vi "WASD Keyboard Drive.vi"() -> (0 "Y-Axis":dbl, 1 "X-Axis":dbl, 2 "key":T1(ring))   [LabVIEW 2012]
uses:
  <vilib>/Utility/inputDevices.llb/keyboardAcquire.vi
  <vilib>/Utility/inputDevices.llb/mouseAcquire.vi
panel:
  in  "Scrolling Down Constant":dbl
  out "Scrolling Down":dbl
  out "button 4":bool
  out "button 3":bool
  out "button 2":bool
  out "button 1":bool
  out "Horizontal Max":dbl
  in  "Scrolling Up Constant":dbl
  out "Vertical":dbl
  out "Horizontal":dbl
  out "Scrolling Up":dbl
  in  "mouse":bool
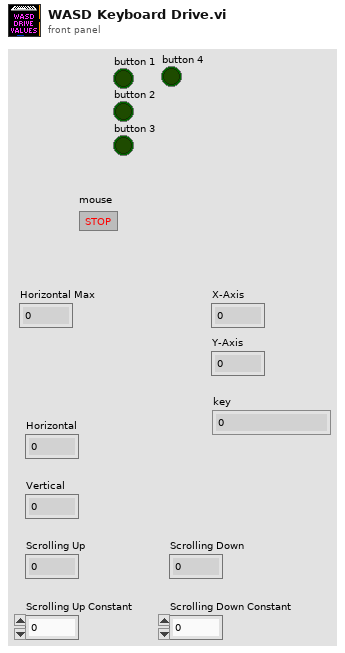
[diagram p1: front panel]
types:
  T1 = enum16{"0", "1", "2", "3", "4", "5", "6", "7", "8", "9", "A", "B", "C", "D", "E", "F", "G", "H", "I", "J", "K", "L", "M", "N", "O", "P", "Q", "R", "S", "T", "U", "V", "W", "X", "Y", "Z", "F1", "F2", "F3", "F4", "F5", "F6", "F7", "F8", "F9", "F10", "F11", "F12", "F13", "F14", "F15", "ADD", "BACK", "BACKSLASH", "CAPITAL", "COMMA", "DECIMAL", "DELETE", "DIVIDE", "DOWN", "END", "EQUALS", "ESCAPE", "GRAVE (`)", "HOME", "INSERT", "LBRACKET", "LCONTROL", "LEFT", "L ALT", "LSHIFT", "LWIN", "MINUS", "MULTIPLY", "NEXT", "NUMLOCK", "NUMPAD_0", "NUMPAD_1", "NUMPAD_2", "NUMPAD_3", "NUMPAD_4", "NUMPAD_5", "NUMPAD_6", "NUMPAD_7", "NUMPAD_8", "NUMPAD_9", "PAUSE", "PERIOD", "PRIOR (PG UP)", "RBRACKET", "RCONTROL", "RETURN", "RIGHT", "R ALT", "RSHIFT", "RWIN", "SCROLL", "SEMICOLON", "SLASH", "SPACE", "SUBTRACT", "TAB", "UP", "ENTER (num pad)", "' (quote)"}
  T2 = cluster{"Horizontal":i32, "Vertical":i32, "Scrolling":i32}
  T3 = cluster{"button 1":bool, "button 2":bool, "button 3":bool, "button 4":bool}
  T4 = enum16{"0", "1", "2", "3", "4", "5", "6", "7", "8", "9", "A", "B", "C", "D", "E", "F", "G", "H", "I", "J", "K", "L", "M", "N", "O", "P", "Q", "R", "S", "T", "U", "V", "W", "X", "Y", "Z", "F1", "F2", "F3", "F4", "F5", "F6", "F7", "F8", "F9", "F10", "F11", "F12", "F13", "F14", "F15", "ADD", "BACK", "BACKSLASH", "CAPITAL", "COMMA", "DECIMAL", "DELETE", "DIVIDE", "DOWN", "END", "EQUALS", "ESCAPE", "GRAVE (`)", "HOME", "INSERT", "LBRACKET", "LCONTROL", "LEFT", "L ALT", "LSHIFT", "LWIN", "MINUS", "MULTIPLY", "NEXT", "NUMLOCK", "NUMPAD_0", "NUMPAD_1", "NUMPAD_2", "NUMPAD_3", "NUMPAD_4", "NUMPAD_5", "NUMPAD_6", "NUMPAD_7", "NUMPAD_8", "NUMPAD_9", "PAUSE", "PERIOD", "PRIOR (PG UP)", "RBRACKET", "RCONTROL", "RETURN", "RIGHT", "R ALT", "RSHIFT", "RWIN", "SCROLL", "SEMICOLON", "SLASH", "SPACE", "SUBTRACT", "TAB", "UP", "ENTER (num pad)", "' (quote)"}[]
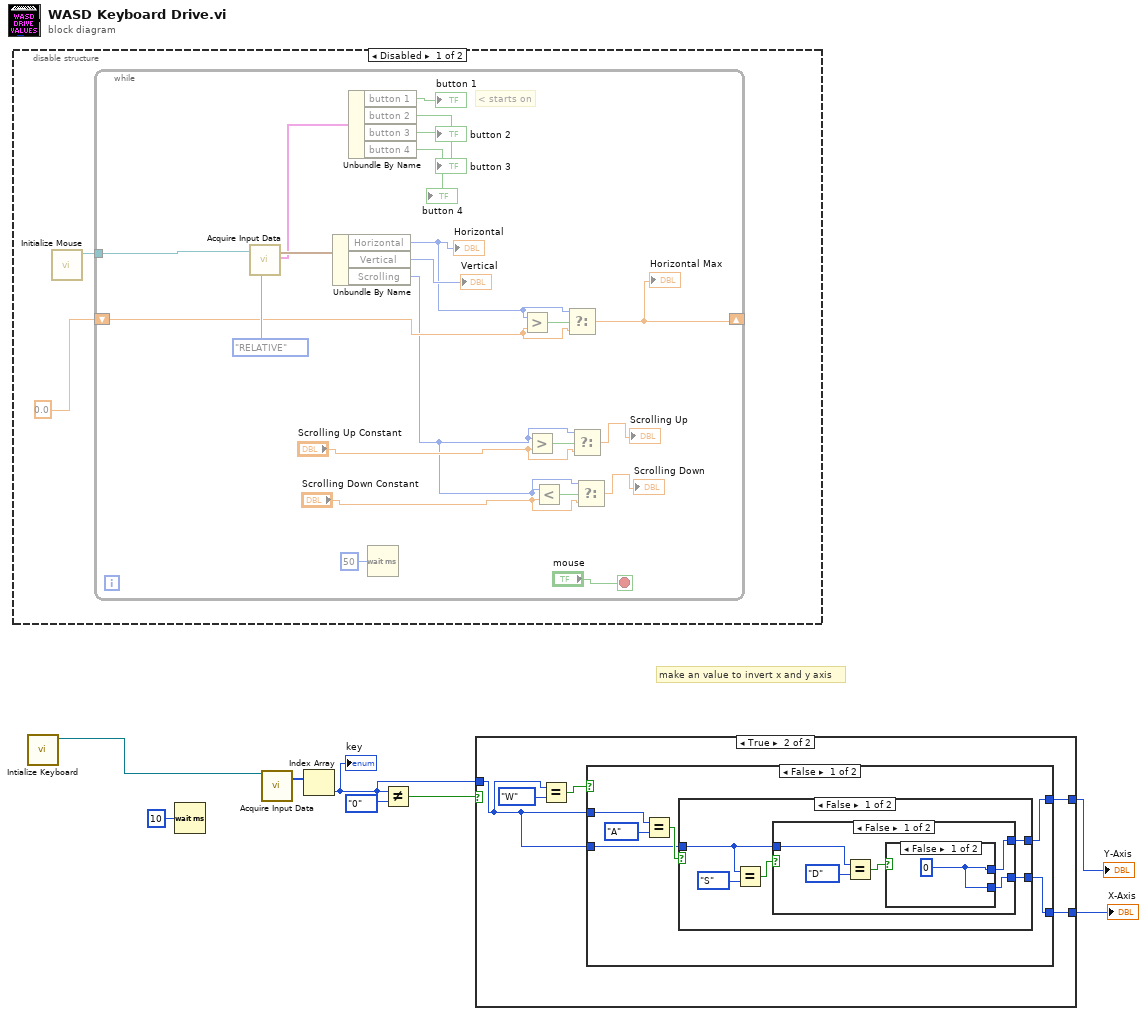
[diagram p0: block diagram]
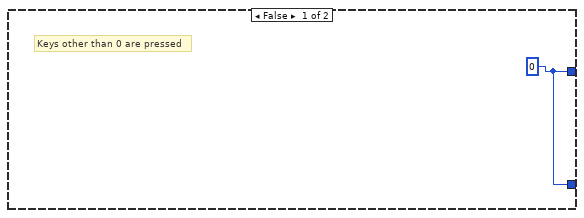
[diagram p2: hidden frame]
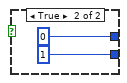
[diagram p3: hidden frame]
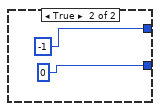
[diagram p4: hidden frame]
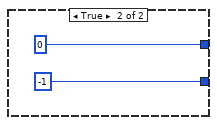
[diagram p5: hidden frame]
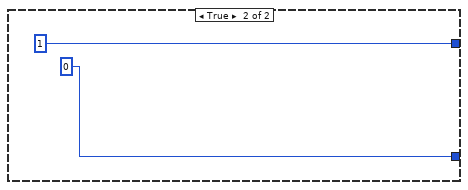
[diagram p6: hidden frame]
diagram:
  # "make an value to invert x and y axis"
  n1 = disable-structure shown="Disabled" {
    frame Disabled {
      n2 = call <vilib>:"Initialize Mouse.vi"() -> ("device ID"=w9:refnum<k1>)  [unwired: 10 in, 1 out]
      n3 = while {
        shift-right: [w20] -> _
        shift-left: 0.0 -> [w21]
        tunnel: w9 -> [w24]
        stop <- "mouse" stop-if-true
        # "< starts on"
        n4 = call-poly <vilib>:"Acquire Input Data.vi"("device ID"=w24, "key mode"=enum16{"RELATIVE", "ABSOLUTE"}."RELATIVE") -> ("axis info"=w25:T2, "button info"=w19:T3)  [unwired: 14 in, 2 out]
        n5 = Unbundle By Name(w25) -> ("Horizontal"=w22:i32, "Vertical"=→"Vertical":i32, "Scrolling"=w12:i32)
        "Horizontal" <- w22
        n6 = Unbundle By Name(w19) -> ("button 1"=→"button 1":bool, "button 2"=→"button 2":bool, "button 3"=→"button 3":bool, "button 4"=→"button 4":bool)
        n7 = Wait (ms)(milliseconds to wait=u32 50) -> ()  [unwired: 1 out]
        n8 = Greater?(x=w22, y=w21) -> (0:w23:bool)
        n9 = Greater?(x=w12, y="Scrolling Up Constant") -> (0:w29:bool)
        n10 = Less?(x=w12, y="Scrolling Down Constant") -> (x < y?=w13:bool)
        n11 = Select(t=w22, s=w23, f=w21) -> (s? t:f=w20:dbl)
        "Horizontal Max" <- w20
        n12 = Select(t=w12, s=w29, f="Scrolling Up Constant") -> (s? t:f=→"Scrolling Up":dbl)
        n13 = Select(t=w12, s=w13, f="Scrolling Down Constant") -> (s? t:f=→"Scrolling Down":dbl)
      }
    }
    frame Enabled {
    }
  }
  n14 = call <vilib>:"Intialize Keyboard.vi"() -> ("device ID"=w8:refnum<k1>)  [unwired: 10 in, 1 out]
  n15 = Wait (ms)(milliseconds to wait=u32 10) -> ()  [unwired: 1 out]
  n16 = call-poly <vilib>:"Acquire Input Data.vi"("device ID"=w8) -> ("keys pressed"=w6:T4)  [unwired: 16 in, 2 out]
  n17 = Index Array(array=w6) -> (element=w3:T1)  [unwired: 1 in]
  "key" <- w3
  n18 = Not Equal?(x=w3, y=T1."0") -> (x != y?=w4:bool)
  n19 = case shown="True" w4 {
    tunnel: w3 -> [_ w35]
    tunnel: [w33 w36] -> w2
    tunnel: [w33 w34] -> w1
    frame False {
      w33 = 0
      # "Keys other than 0 are pressed"
    }
    frame True {
      n20 = Equal?(x=w35, y=T1."W") -> (x = y?=w37:bool)
      n21 = case shown="False" w37 {
        tunnel: [w40 1] -> w36
        tunnel: w35 -> [w43 _]
        tunnel: w35 -> [w41 _]
        tunnel: [w39 0] -> w34
        frame False {
          n22 = Equal?(x=w43, y=T1."A") -> (x = y?=w42:bool)
          n23 = case shown="False" w42 {
            tunnel: w41 -> [w47 _]
            tunnel: [w46 0] -> w40
            tunnel: [w45 -1] -> w39
            frame False {
              n24 = Equal?(x=w47, y=T1."S") -> (x = y?=w48:bool)
              n25 = case shown="False" w48 {
                tunnel: w47 -> [w53 _]
                tunnel: [w51 -1] -> w46
                tunnel: [w50 0] -> w45
                frame False {
                  n26 = Equal?(x=w53, y=T1."D") -> (x = y?=w52:bool)
                  n27 = case shown="False" w52 {
                    tunnel: [w55 0] -> w51
                    tunnel: [w55 1] -> w50
                    frame False {
                      w55 = 0
                    }
                    frame True {
                    }
                  }
                }
                frame True {
                }
              }
            }
            frame True {
            }
          }
        }
        frame True {
        }
      }
    }
  }
  "Y-Axis" <- w2
  "X-Axis" <- w1
